vi "PWM Input User Interface.vi"() -> ()   [LabVIEW 2023, in "GUI.lvlib" / "Diagnostic.lvlib"]
uses:
  Diagnostic.lvlib
  Control/PWM Input 6345.ctl
  Control/PWM Input.ctl
  Control/PWM Input 6363.ctl
  Control/PWM Input 6612.ctl
  HardwareAbstractionLayer_LVOOP/PWM Input/NI PWM Input_class/NI PWM Input.lvclass
  D:/eDCU LTT/VT LTT Project/Source Code/HardwareAbstractionLayer_LVOOP/PWM Input/PWM Input_class/PWM Input.lvclass
  HardwareAbstractionLayer_LVOOP/Database/SQL Public VI/Control/DB Options.ctl
  HardwareAbstractionLayer_LVOOP/Main/Class Ref.ctl
  HardwareAbstractionLayer_LVOOP/DMM/DMM.lvclass
  HardwareAbstractionLayer_LVOOP/Function Generator/Function Generator.lvclass
  HardwareAbstractionLayer_LVOOP/Oscilloscope/Oscilloscope.lvclass
  HardwareAbstractionLayer_LVOOP/PowerSupply/PowerSupply.lvclass
  HardwareAbstractionLayer_LVOOP/Teststand/Teststand.lvclass
  HardwareAbstractionLayer_LVOOP/Analog Output/AO/AO.lvclass
  HardwareAbstractionLayer_LVOOP/Analog Input/AI/AI.lvclass
  HardwareAbstractionLayer_LVOOP/Database/Database.lvclass
  HardwareAbstractionLayer_LVOOP/Digital Output/DO_class/DO.lvclass
  HardwareAbstractionLayer_LVOOP/Digital Input/DI_class/DI.lvclass
  HardwareAbstractionLayer_LVOOP/PWM Output/PWM Output_class/PWM Output.lvclass
  HardwareAbstractionLayer_LVOOP/PWM Input/PWM Input_class/PWM Input.lvclass
  HardwareAbstractionLayer_LVOOP/NI Switch/NISwitch_class/NISwitch.lvclass
  HardwareAbstractionLayer_LVOOP/Modbus/Modbus_class/Modbus.lvclass
  HardwareAbstractionLayer_LVOOP/CAN/CAN Lib/CAN_class/CAN.lvclass
  HardwareAbstractionLayer_LVOOP/Main/Main.lvclass
panel:
  in  "Stop Acquire":bool
  in  "Start Acquire":bool
  out "error out":errorcluster
  in  "error in":errorcluster
  in  "Operation":T1(tab)
  in  "PXIe - 6345":T2 {"Channel 3"."Duty Cycle" format="%.3g"; "Channel 3"."Frequency" format="%.3g"; "Channel 2"."Duty Cycle" format="%.3g"; "Channel 2"."Frequency" format="%.3g"; "Channel 1"."Duty Cycle" format="%.3g"; "Channel 1"."Frequency" format="%.3g"; "Channel 0"."Duty Cycle" format="%.3g"; "Channel 0"."Frequency" format="%.3g"}
  in  "PXIe - 6363":T4 {"Channel 3"."Duty Cycle" format="%.3g"; "Channel 3"."Frequency" format="%.3g"; "Channel 2"."Duty Cycle" format="%.3g"; "Channel 2"."Frequency" format="%.3g"; "Channel 1"."Duty Cycle" format="%.3g"; "Channel 1"."Frequency" format="%.3g"; "Channel 0"."Duty Cycle" format="%.3g"; "Channel 0"."Frequency" format="%.3g"}
  in  "PXIe - 6612 M1":T5 {"Channel 0"."Duty Cycle" format="%.3g"; "Channel 0"."Frequency" format="%.3g"; "Channel 7"."Duty Cycle" format="%.3g"; "Channel 7"."Frequency" format="%.3g"; "Channel 6"."Duty Cycle" format="%.3g"; "Channel 6"."Frequency" format="%.3g"; "Channel 5"."Duty Cycle" format="%.3g"; "Channel 5"."Frequency" format="%.3g"; "Channel 4"."Duty Cycle" format="%.3g"; "Channel 4"."Frequency" format="%.3g"; "Channel 3"."Duty Cycle" format="%.3g"; "Channel 3"."Frequency" format="%.3g"; "Channel 2"."Duty Cycle" format="%.3g"; "Channel 2"."Frequency" format="%.3g"; "Channel 1"."Duty Cycle" format="%.3g"; "Channel 1"."Frequency" format="%.3g"}
  in  "PXIe - 6612 M2":T5 {"Channel 0"."Duty Cycle" format="%.3g"; "Channel 0"."Frequency" format="%.3g"; "Channel 7"."Duty Cycle" format="%.3g"; "Channel 7"."Frequency" format="%.3g"; "Channel 6"."Duty Cycle" format="%.3g"; "Channel 6"."Frequency" format="%.3g"; "Channel 5"."Duty Cycle" format="%.3g"; "Channel 5"."Frequency" format="%.3g"; "Channel 4"."Duty Cycle" format="%.3g"; "Channel 4"."Frequency" format="%.3g"; "Channel 3"."Duty Cycle" format="%.3g"; "Channel 3"."Frequency" format="%.3g"; "Channel 2"."Duty Cycle" format="%.3g"; "Channel 2"."Frequency" format="%.3g"; "Channel 1"."Duty Cycle" format="%.3g"; "Channel 1"."Frequency" format="%.3g"}
  in  "Stop":bool caption="Blank"
  # "Frequency"
  # "Dutycycles"
  # "PWM Input"
  # "Device:"
  # "***Note:  Duty Cycle Max Values Is 0.99 Only"
  # "Frequency"
  # "Dutycycles"
  # "Terminal Configuration"
  # "Enabled"
  # "Physical Channel"
  # "Frequency"
  # "Dutycycles"
  # "Terminal Configuration"
  # "Enabled"
  # "Physical Channel"
  # "Frequency"
  # "Dutycycles"
  # "Terminal Configuration"
  # "Enabled"
  # "Physical Channel"
  # "Frequency"
  # "Dutycycles"
  # "Enabled"
  # "Physical Channel"
  # "Terminal Configuration"
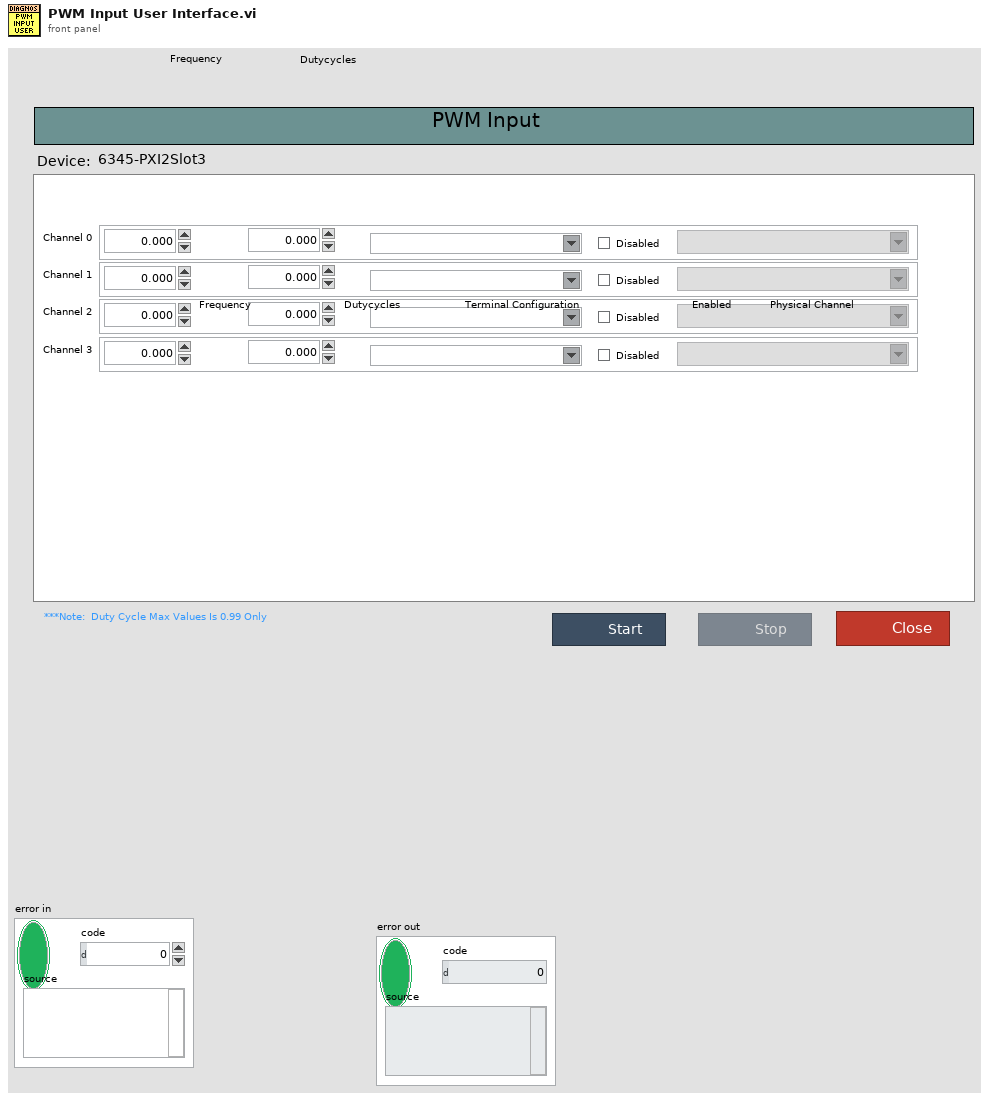
[diagram p1: front panel]
types:
  T1 = enum32{"6345-PXI2Slot3", "6363-PXI2Slot2", "6612-PXI2Slot7", "6612-PXI2Slot8"}
  T2 = typedef "GUI.lvlib/Diagnostic.lvlib/PWM Input 6345.ctl" = cluster{"Channel 0":T3, "Channel 1":T3, "Channel 2":T3, "Channel 3":T3}
  T3 = typedef "GUI.lvlib/Diagnostic.lvlib/PWM Input.ctl" = cluster{"Frequency":dbl, "Duty Cycle":dbl, "DAQmx Terminal":tag, "Checkbox":bool, "DAQmx Physical Channel":tag}
  T4 = typedef "GUI.lvlib/Diagnostic.lvlib/PWM Input 6363.ctl" = cluster{"Channel 0":T3, "Channel 1":T3, "Channel 2":T3, "Channel 3":T3}
  T5 = typedef "GUI.lvlib/Diagnostic.lvlib/PWM Input 6612.ctl" = cluster{"Channel 0":T3, "Channel 1":T3, "Channel 2":T3, "Channel 3":T3, "Channel 4":T3, "Channel 5":T3, "Channel 6":T3, "Channel 7":T3}
  T6 = typedef "HardwareAbstractionLayer_LVOOP.lvlib/Database.lvclass/DB Options.ctl" = enum16{"Init", "Select Data", "Insert Data", "Update Data", "Delete Data", "Execute Query", "Create Schema", "Create Table", "List Tables", "List Columns", "Close"}
  T7 = typedef "HardwareAbstractionLayer_LVOOP.lvlib/Main.lvclass/Class Ref.ctl" = cluster{"DMM":refnum<class "DMM.lvclass">, "Function Generator":refnum<class "Function Generator.lvclass">, "Oscilloscope":refnum<class "Oscilloscope.lvclass">, "PowerSupply":refnum<class "PowerSupply.lvclass">, "Teststand":refnum<class "Teststand.lvclass">, "AO":refnum<class "AO.lvclass">, "AI":refnum<class "AI.lvclass">, "Database":refnum<class "Database.lvclass">, "AO Waveform Generation":refnum<class "AO.lvclass">, "DO":refnum<class "DO.lvclass">, "DI":refnum<class "DI.lvclass">, "PWM Output":refnum<class "PWM Output.lvclass">, "PWM Input":refnum<class "PWM Input.lvclass">, "RelayOutput":refnum<class "NISwitch.lvclass">, "Modbus":refnum<class "Modbus.lvclass">, "CAN":refnum<class "CAN.lvclass">}
  T8 = enum8{"Enabled", "Disabled", "Disabled and Grayed Out"}
  T9 = cluster{"Value[0]":T3, "Value[1]":T3, "Value[2]":T3, "Value[3]":T3}
  T10 = cluster{"[0]":T3, "[1]":T3, "[2]":T3, "[3]":T3, "[4]":T3, "[5]":T3, "[6]":T3, "[7]":T3}
  T11 = cluster{"Channel 0":T3, "Channel 1":T3, "Channel 2":T3, "Channel 3":T3, "Channel 4":T3, "Channel 5":T3, "Channel 6":T3, "Channel 7":T3}
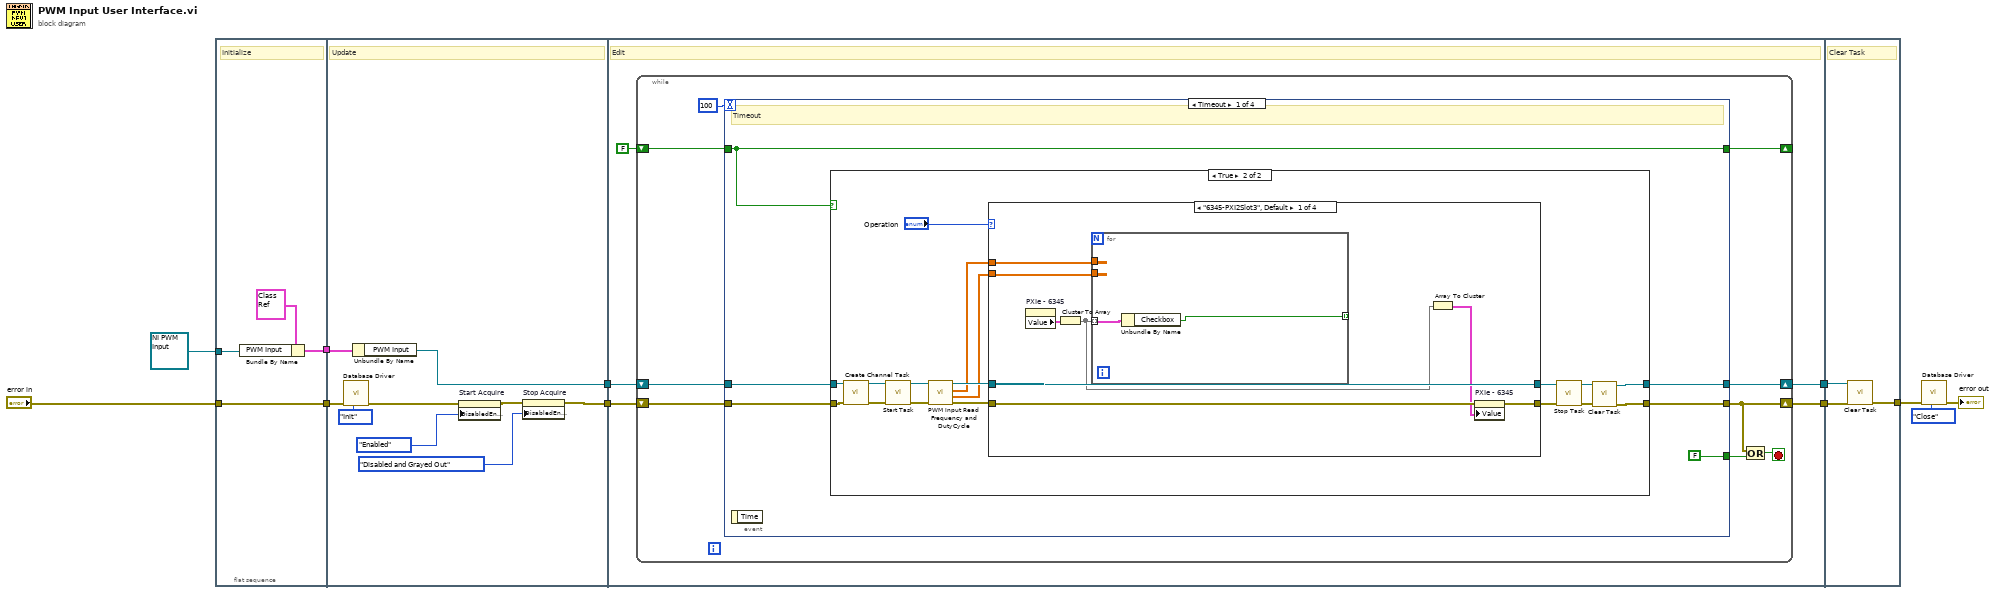
[diagram p0: block diagram]
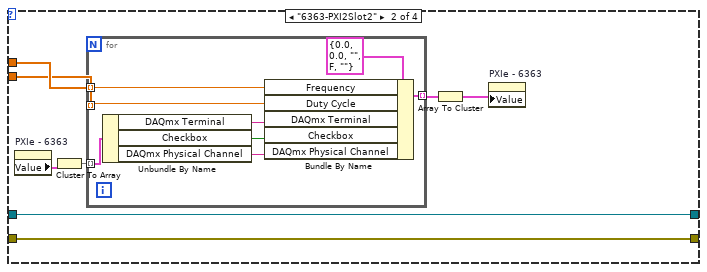
[diagram p3: hidden frame]
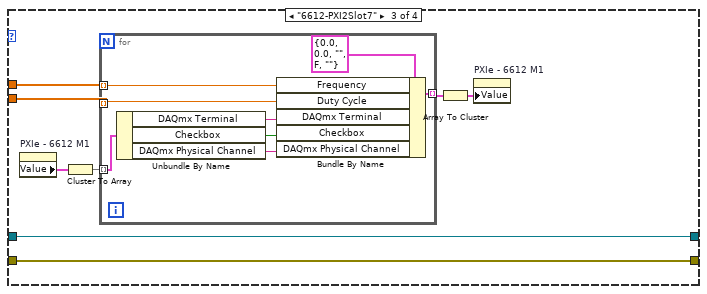
[diagram p4: hidden frame]
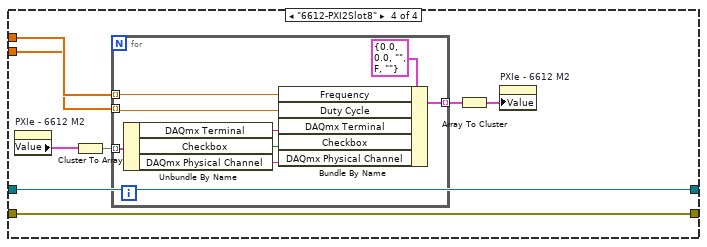
[diagram p5: hidden frame]
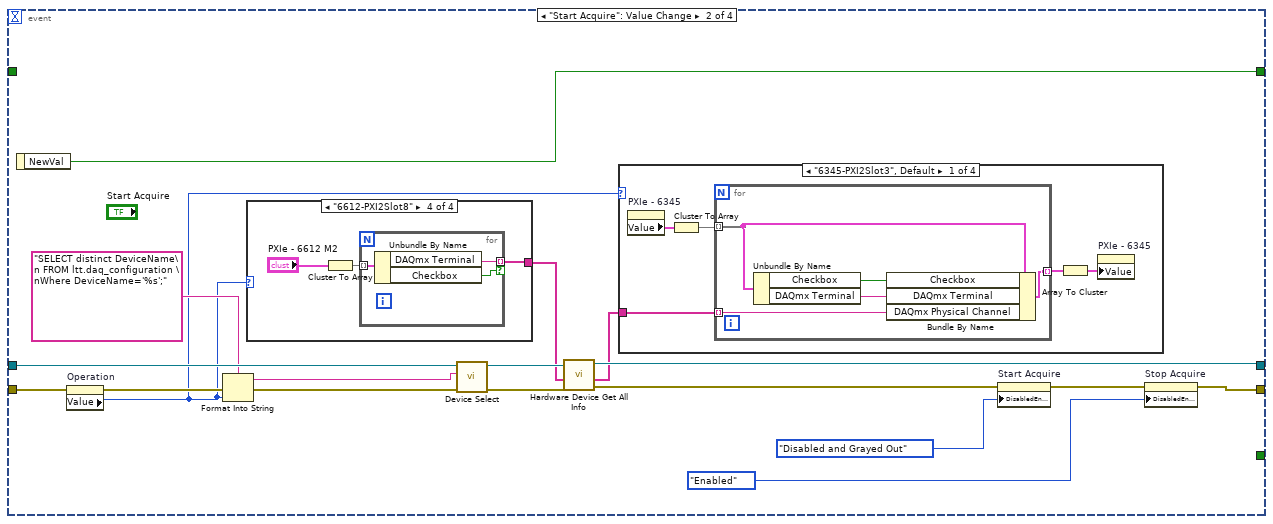
[diagram p6: hidden frame]
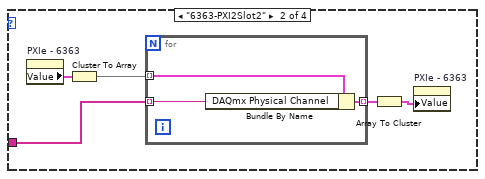
[diagram p7: hidden frame]
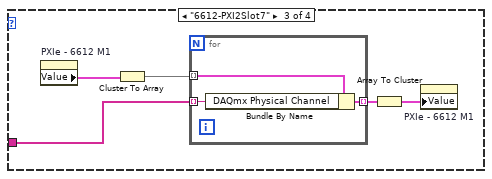
[diagram p8: hidden frame]
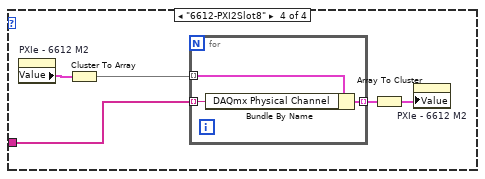
[diagram p9: hidden frame]
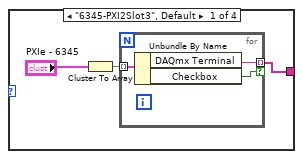
[diagram p10: hidden frame]
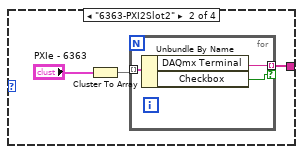
[diagram p11: hidden frame]
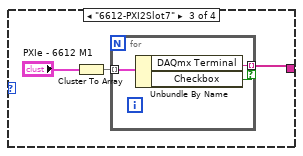
[diagram p12: hidden frame]
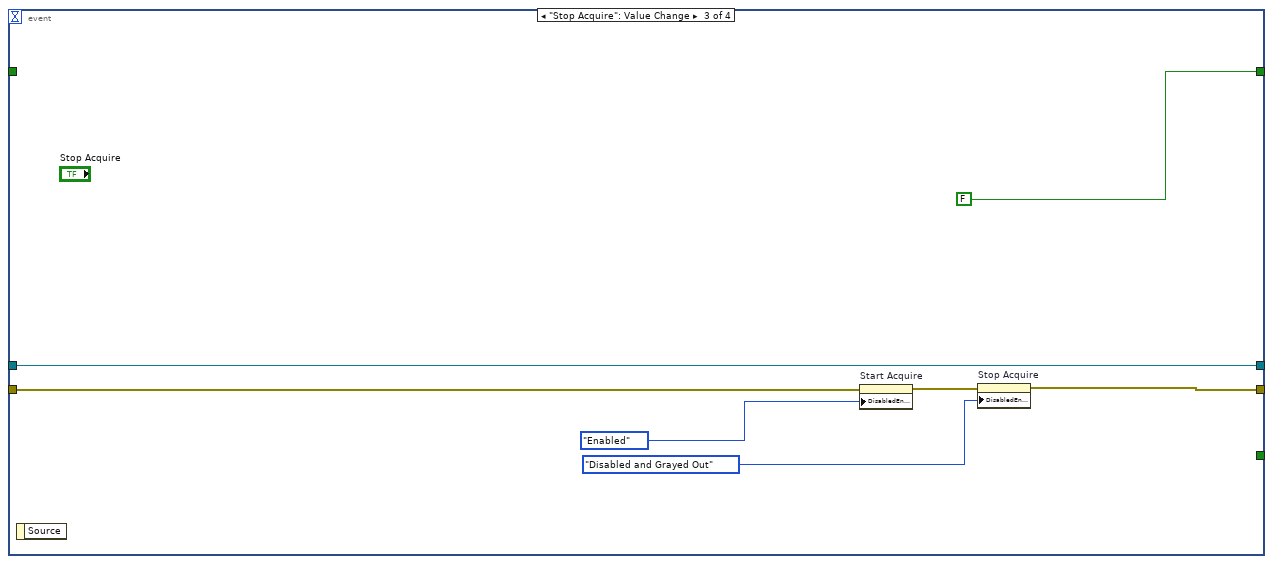
[diagram p13: hidden frame]
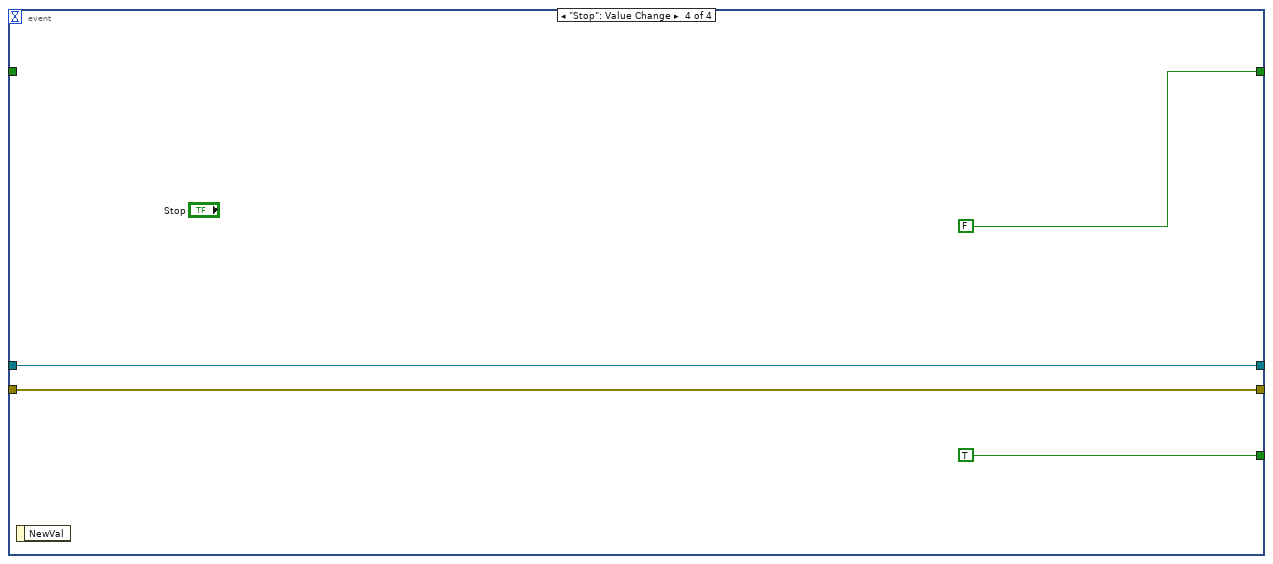
[diagram p14: hidden frame]
diagram:
  n1 = flat-sequence {
    tunnel: [w15] -> w11
    tunnel: "error in" -> [w15]
    tunnel: refnum<class "NI PWM Input.lvclass"> refnum ("HardwareAbstractionLayer_LVOOP.lvlib:NI PWM Input.lvclass") -> [w13]
    tunnel: [w12] -> w9
    tunnel: w11 -> [w23]
    tunnel: [w18] -> w10
    tunnel: w9 -> [w24]
    tunnel: [w21] -> w8
    tunnel: w10 -> [w29]
    tunnel: w8 -> [w27]
    tunnel: [w28] -> w7
    tunnel: [w26] -> w5
    tunnel: w7 -> [w211]
    tunnel: w5 -> [w210]
    tunnel: [w209] -> w4
    frame #0 {
      # "Initialize"
      n2 = Bundle By Name(cluster=T7 {"DMM"=refnum, "Function Generator"=refnum, "Oscilloscope"=refnum, "PowerSupply"=refnum, "Teststand"=refnum, "AO"=refnum, "AI"=refnum, "Database"=refnum, "AO Waveform Generation"=refnum, "DO"=refnum, "DI"=refnum, "PWM Output"=refnum, "PWM Input"=refnum, "RelayOutput"=refnum, "Modbus"=refnum, "CAN"=refnum} ("Class Cluster"), "PWM Input"=w13) -> (w12:T7)
    }
    frame #1 {
      # "Update"
      n3 = call "Database Driver.vi"("Options"=DB_Options."Init", "error in"=w23) -> ("error out"=w20:errorcluster)  [unwired: 6 in, 3 out]
      n4 = Unbundle By Name(w24) -> ("PWM Input"=w21:refnum<class "PWM Input.lvclass">)
      n5 = property on="Start Acquire" class="Bool"(error in=w20, "DisabledEnum"=T8."Enabled" ("Disabled")) -> (error out=w19:errorcluster)  [unwired: 1 in, 1 out]
      n6 = property on="Stop Acquire" class="Bool"(error in=w19, "DisabledEnum"=T8."Disabled and Grayed Out" ("Disabled")) -> (error out=w18:errorcluster)  [unwired: 1 in, 1 out]
    }
    frame #2 {
      # "Edit"
      n7 = while {
        shift-right: [w30] -> w28
        shift-left: w29 -> [w36]
        shift-right: [w34] -> w26
        shift-left: w27 -> [w35]
        shift-right: [w33] -> _
        shift-left: FALSE ("NewVal") -> [w32]
        stop <- w31 stop-if-true
        n8 = event shown="[0] Timeout" {
          selector: _ -> [_ _ _ _]
          dyn-events: _ -> [_ _ _ _]
          timeout: 100 -> [_ _ _ _]
          tunnel: [FALSE ("Stop") _ _ TRUE ("Stop")] -> w37
          tunnel: w36 -> [w44 w139 w203 w206]
          tunnel: [w43 w128 w199 w206] -> w30
          tunnel: [w42 w125 w204 w207] -> w34
          tunnel: w35 -> [w41 w137 w204 w207]
          tunnel: [w39 w127 FALSE ("NewVal") FALSE ("NewVal")] -> w33
          tunnel: w32 -> [w39 _ _ _]
          event Timeout {
            # "Timeout"
            n9 = event-data() -> ()  [unwired: 1 in, 1 out]
            n10 = case shown="True" w39 {
              tunnel: w44 -> [w45 w47]
              tunnel: [w45 w49] -> w43
              tunnel: [w46 w52] -> w42
              tunnel: w41 -> [w46 w48]
              frame False {
              }
              frame True {
                n11 = call-dynamic "Create Channel Task.vi"("error in (no error)"=w47, "PWM Input in"=w48) -> ("error out"=w57:errorcluster, "PWM Input out"=w58:refnum<class "PWM Input.lvclass">)  [unwired: 8 in]
                n12 = call-dynamic "Start Task.vi"("error in (no error)"=w57, "PWM Input in"=w58) -> ("error out"=w56:errorcluster, "PWM Input out"=w55:refnum<class "PWM Input.lvclass">)  [unwired: 8 in]
                n13 = call-dynamic "PWM Input Read Frequency and DutyCycle.vi"("error in (no error)"=w56, "PWM Input in"=w55) -> ("error out"=w60:errorcluster, "Duty Cycle"=w59:dbl[], "Frequency"=w61:dbl[], "PWM Input out"=w62:refnum<class "PWM Input.lvclass">)  [unwired: 6 in]
                n14 = case shown="\"6345-PXI2Slot3\", Default" "Operation" {
                  tunnel: w60 -> [w68 w80 w96 w112]
                  tunnel: [w67 w80 w96 w112] -> w51
                  tunnel: [w71 w81 w97 w113] -> w54
                  tunnel: w62 -> [w71 w81 w97 w113]
                  tunnel: w61 -> [w70 w78 w94 w111]
                  tunnel: w59 -> [w69 w77 w93 w110]
                  frame "6345-PXI2Slot3", Default {
                    n15 = property on="PXIe - 6345" class="Clust (strict)"() -> ("Value"=w65:T2)  [unwired: 2 in, 2 out]
                    n16 = Cluster To Array(cluster=w65) -> (array=w64:T3[])
                    n17 = for {
                      tunnel: w70 -> [_]
                      tunnel: w69 -> [_]
                      tunnel: w64 -> [w73] mode=indexing
                      tunnel: [w72] -> _ mode=indexing
                      n18 = Unbundle By Name(w73) -> ("Checkbox"=w72:bool)
                    }
                    n19 = Array To Cluster(array=w64) -> (cluster=w66:T9)
                    n20 = property on="PXIe - 6345" class="Clust (strict)"(error in=w68, "Value"=w66) -> (error out=w67:errorcluster)  [unwired: 1 in, 1 out]
                  }
                  frame "6363-PXI2Slot2" {
                    n21 = property on="PXIe - 6363" class="Clust (strict)"() -> ("Value"=w75:T4)  [unwired: 2 in, 2 out]
                    n22 = Cluster To Array(cluster=w75) -> (array=w76:T3[])
                    n23 = for {
                      tunnel: w78 -> [w87] mode=indexing
                      tunnel: w77 -> [w88] mode=indexing
                      tunnel: [w86] -> w79 mode=indexing
                      tunnel: w76 -> [w85] mode=indexing
                      n24 = Unbundle By Name(w85) -> ("DAQmx Terminal"=w84:tag, "Checkbox"=w83:bool, "DAQmx Physical Channel"=w82:tag)
                      n25 = Bundle By Name(cluster=T3 {"Frequency"=0.0, "Duty Cycle"=0.0, "DAQmx Terminal"="", "Checkbox"=FALSE, "DAQmx Physical Channel"=""} ("PWM Input"), "Frequency"=w87, "Duty Cycle"=w88, "DAQmx Terminal"=w84, "Checkbox"=w83, "DAQmx Physical Channel"=w82) -> (w86:T3)
                    }
                    n26 = Array To Cluster(array=w79) -> (cluster=w74:cluster{"[0]":T3, "[1]":T3, "[2]":T3, "[3]":T3})
                    n27 = property on="PXIe - 6363" class="Clust (strict)"("Value"=w74) -> ()  [unwired: 2 in, 2 out]
                  }
                  frame "6612-PXI2Slot7" {
                    n28 = property on="PXIe - 6612 M1" class="Clust (strict)"() -> ("Value"=w91:T5)  [unwired: 2 in, 2 out]
                    n29 = Cluster To Array(cluster=w91) -> (array=w90:T3[])
                    n30 = for {
                      tunnel: w94 -> [w103] mode=indexing
                      tunnel: w93 -> [w104] mode=indexing
                      tunnel: [w102] -> w95 mode=indexing
                      tunnel: w90 -> [w101] mode=indexing
                      n31 = Unbundle By Name(w101) -> ("DAQmx Terminal"=w100:tag, "Checkbox"=w99:bool, "DAQmx Physical Channel"=w98:tag)
                      n32 = Bundle By Name(cluster=T3 {"Frequency"=0.0, "Duty Cycle"=0.0, "DAQmx Terminal"="", "Checkbox"=FALSE, "DAQmx Physical Channel"=""} ("PWM Input"), "Frequency"=w103, "Duty Cycle"=w104, "DAQmx Terminal"=w100, "Checkbox"=w99, "DAQmx Physical Channel"=w98) -> (w102:T3)
                    }
                    n33 = Array To Cluster(array=w95) -> (cluster=w92:T10)
                    n34 = property on="PXIe - 6612 M1" class="Clust (strict)"("Value"=w92) -> ()  [unwired: 2 in, 2 out]
                  }
                  frame "6612-PXI2Slot8" {
                    n35 = property on="PXIe - 6612 M2" class="Clust (strict)"() -> ("Value"=w107:T11)  [unwired: 2 in, 2 out]
                    n36 = Cluster To Array(cluster=w107) -> (array=w108:T3[])
                    n37 = for {
                      tunnel: w111 -> [w119] mode=indexing
                      tunnel: w110 -> [w120] mode=indexing
                      tunnel: [w118] -> w109 mode=indexing
                      tunnel: w108 -> [w117] mode=indexing
                      n38 = Unbundle By Name(w117) -> ("DAQmx Terminal"=w116:tag, "Checkbox"=w115:bool, "DAQmx Physical Channel"=w114:tag)
                      n39 = Bundle By Name(cluster=T3 {"Frequency"=0.0, "Duty Cycle"=0.0, "DAQmx Terminal"="", "Checkbox"=FALSE, "DAQmx Physical Channel"=""} ("PWM Input"), "Frequency"=w119, "Duty Cycle"=w120, "DAQmx Terminal"=w116, "Checkbox"=w115, "DAQmx Physical Channel"=w114) -> (w118:T3)
                    }
                    n40 = Array To Cluster(array=w109) -> (cluster=w106:T10)
                    n41 = property on="PXIe - 6612 M2" class="Clust (strict)"("Value"=w106) -> ()  [unwired: 2 in, 2 out]
                  }
                }
                n42 = call-dynamic "Stop Task.vi"("error in (no error)"=w51, "PWM Input in"=w54) -> ("error out"=w50:errorcluster, "PWM Input out"=w53:refnum<class "PWM Input.lvclass">)  [unwired: 8 in]
                n43 = call-dynamic "Clear Task.vi"("error in (no error)"=w50, "PWM Input in"=w53) -> ("error out"=w49:errorcluster, "PWM Input out"=w52:refnum<class "PWM Input.lvclass">)  [unwired: 8 in]
              }
            }
          }
          event "Start Acquire": Value Change {
            n44 = event-data() -> ("NewVal"=w127:bool)  [unwired: 1 in]
            n45 = property on="Operation" class="TabCtl (strict)"(error in=w139) -> (error out=w138:errorcluster, "Value"=w123:T1)  [unwired: 1 in, 1 out]
            n46 = Format Into String(format string="SELECT distinct DeviceName\n FROM ltt.daq_configuration \nWhere DeviceName='%s';" ("SQL query"), error in=w138, w123) -> (resulting string=w134:string, error out=w136:errorcluster)  [unwired: 1 in]
            n47 = case shown="\"6612-PXI2Slot8\"" w123 {
              tunnel: [w174 w180 w186 w192] -> w126
              frame "6345-PXI2Slot3", Default {
                n48 = Cluster To Array(cluster="PXIe - 6345") -> (array=w176:T3[])
                n49 = for {
                  tunnel: w176 -> [w179] mode=indexing
                  tunnel: [w178] -> w174 mode=indexing if=w177
                  n50 = Unbundle By Name(w179) -> ("DAQmx Terminal"=w178:tag, "Checkbox"=w177:bool)
                }
              }
              frame "6363-PXI2Slot2" {
                n51 = Cluster To Array(cluster="PXIe - 6363") -> (array=w181:T3[])
                n52 = for {
                  tunnel: w181 -> [w185] mode=indexing
                  tunnel: [w184] -> w180 mode=indexing if=w183
                  n53 = Unbundle By Name(w185) -> ("DAQmx Terminal"=w184:tag, "Checkbox"=w183:bool)
                }
              }
              frame "6612-PXI2Slot7" {
                n54 = Cluster To Array(cluster="PXIe - 6612 M1") -> (array=w187:T3[])
                n55 = for {
                  tunnel: [w191] -> w186 mode=indexing if=w190
                  tunnel: w187 -> [w189] mode=indexing
                  n56 = Unbundle By Name(w189) -> ("DAQmx Terminal"=w191:tag, "Checkbox"=w190:bool)
                }
              }
              frame "6612-PXI2Slot8" {
                n57 = Cluster To Array(cluster="PXIe - 6612 M2") -> (array=w193:T3[])
                n58 = for {
                  tunnel: w193 -> [w197] mode=indexing
                  tunnel: [w196] -> w192 mode=indexing if=w195
                  n59 = Unbundle By Name(w197) -> ("DAQmx Terminal"=w196:tag, "Checkbox"=w195:bool)
                }
              }
            }
            n60 = call-dynamic "Device Select.vi"("error in (no error)"=w136, "SQL query"=w134, "PWM Input in"=w137) -> ("error out"=w133:errorcluster, "PWM Input out"=w132:refnum<class "PWM Input.lvclass">)  [unwired: 7 in]
            n61 = call-dynamic "Hardware Device Get All Info.vi"("error in (no error)"=w133, "Terminals"=w126, "PWM Input in"=w132) -> ("error out"=w124:errorcluster, "CI.PhysicalChans"=w122:tag[], "PWM Input out"=w125:refnum<class "PWM Input.lvclass">)  [unwired: 6 in]
            n62 = case shown="\"6345-PXI2Slot3\", Default" w123 {
              tunnel: w122 -> [w140 w153 w161 w169]
              frame "6345-PXI2Slot3", Default {
                n63 = property on="PXIe - 6345" class="Clust (strict)"() -> ("Value"=w144:T2)  [unwired: 2 in, 2 out]
                n64 = Cluster To Array(cluster=w144) -> (array=w143:T3[])
                n65 = for {
                  tunnel: w143 -> [w147] mode=indexing
                  tunnel: w140 -> [w149] mode=indexing
                  tunnel: [w148] -> w142 mode=indexing
                  n66 = Unbundle By Name(w147) -> ("Checkbox"=w145:bool, "DAQmx Terminal"=w146:tag)
                  n67 = Bundle By Name(cluster=w147, "Checkbox"=w145, "DAQmx Terminal"=w146, "DAQmx Physical Channel"=w149) -> (w148:T3)
                }
                n68 = Array To Cluster(array=w142) -> (cluster=w141:cluster{"[0]":T3, "[1]":T3, "[2]":T3, "[3]":T3})
                n69 = property on="PXIe - 6345" class="Clust (strict)"("Value"=w141) -> ()  [unwired: 2 in, 2 out]
              }
              frame "6363-PXI2Slot2" {
                n70 = property on="PXIe - 6363" class="Clust (strict)"() -> ("Value"=w151:T4)  [unwired: 2 in, 2 out]
                n71 = Cluster To Array(cluster=w151) -> (array=w154:T3[])
                n72 = for {
                  tunnel: w154 -> [w157] mode=indexing
                  tunnel: w153 -> [w156] mode=indexing
                  tunnel: [w155] -> w152 mode=indexing
                  n73 = Bundle By Name(cluster=w157, "DAQmx Physical Channel"=w156) -> (w155:T3)
                }
                n74 = Array To Cluster(array=w152) -> (cluster=w150:cluster{"[0]":T3, "[1]":T3, "[2]":T3, "[3]":T3})
                n75 = property on="PXIe - 6363" class="Clust (strict)"("Value"=w150) -> ()  [unwired: 2 in, 2 out]
              }
              frame "6612-PXI2Slot7" {
                n76 = property on="PXIe - 6612 M1" class="Clust (strict)"() -> ("Value"=w158:T5)  [unwired: 2 in, 2 out]
                n77 = Cluster To Array(cluster=w158) -> (array=w162:T3[])
                n78 = for {
                  tunnel: w162 -> [w165] mode=indexing
                  tunnel: w161 -> [w164] mode=indexing
                  tunnel: [w163] -> w160 mode=indexing
                  n79 = Bundle By Name(cluster=w165, "DAQmx Physical Channel"=w164) -> (w163:T3)
                }
                n80 = Array To Cluster(array=w160) -> (cluster=w159:T10)
                n81 = property on="PXIe - 6612 M1" class="Clust (strict)"("Value"=w159) -> ()  [unwired: 2 in, 2 out]
              }
              frame "6612-PXI2Slot8" {
                n82 = property on="PXIe - 6612 M2" class="Clust (strict)"() -> ("Value"=w167:T5)  [unwired: 2 in, 2 out]
                n83 = Cluster To Array(cluster=w167) -> (array=w170:T3[])
                n84 = for {
                  tunnel: w170 -> [w173] mode=indexing
                  tunnel: w169 -> [w172] mode=indexing
                  tunnel: [w171] -> w168 mode=indexing
                  n85 = Bundle By Name(cluster=w173, "DAQmx Physical Channel"=w172) -> (w171:T3)
                }
                n86 = Array To Cluster(array=w168) -> (cluster=w166:T10)
                n87 = property on="PXIe - 6612 M2" class="Clust (strict)"("Value"=w166) -> ()  [unwired: 2 in, 2 out]
              }
            }
            n88 = property on="Start Acquire" class="Bool"(error in=w124, "DisabledEnum"=T8."Disabled and Grayed Out" ("Disabled")) -> (error out=w129:errorcluster)  [unwired: 1 in, 1 out]
            n89 = property on="Stop Acquire" class="Bool"(error in=w129, "DisabledEnum"=T8."Enabled" ("Disabled")) -> (error out=w128:errorcluster)  [unwired: 1 in, 1 out]
          }
          event "Stop Acquire": Value Change {
            n90 = event-data() -> ()  [unwired: 1 in, 1 out]
            n91 = property on="Start Acquire" class="Bool"(error in=w203, "DisabledEnum"=T8."Enabled" ("Disabled")) -> (error out=w200:errorcluster)  [unwired: 1 in, 1 out]
            n92 = property on="Stop Acquire" class="Bool"(error in=w200, "DisabledEnum"=T8."Disabled and Grayed Out" ("Disabled")) -> (error out=w199:errorcluster)  [unwired: 1 in, 1 out]
          }
          event "Stop": Value Change {
            n93 = event-data() -> ()  [unwired: 1 in, 1 out]
          }
        }
        n94 = Compound Arithmetic op=OR(w30, w37) -> (w31:bool)
      }
    }
    frame #3 {
      # "Clear Task"
      n95 = call-dynamic "Clear Task.vi"("error in (no error)"=w211, "PWM Input in"=w210) -> ("error out"=w209:errorcluster)  [unwired: 8 in, 1 out]
    }
  }
  n96 = call "Database Driver.vi"("Options"=DB_Options."Close", "error in"=w4) -> ("error out"=→"error out":errorcluster)  [unwired: 6 in, 3 out]
